vi "Data_filtering_test_2.vi"() -> ()   [LabVIEW 2018]
uses:
  7127b0f4-44e3-4b60-8031-f21aa20547ce.vi
  7127b0f4-44e3-4b60-8031-f21aa20547ce.vi/98f45aaf-d764-4694-8feb-128a91b70d7c.vi
  <vilib>/Analysis/NI_AALBase.lvlib
  <vilib>/Analysis/NI_AALPro.lvlib
panel:
  out "SD speed 2":dbl format="%0.2f"
  out "SD speed 1":dbl format="%0.2f"
  out "SD ideal speed 2":dbl format="%0.2f"
  out "SD ideal speed 1":dbl format="%0.2f"
  out "Speed 2":dbl format="%0.2f"
  out "Speed 1":dbl format="%0.2f"
  out "Ideal speed 2":dbl format="%0.2f"
  out "Ideal speed 1":dbl format="%0.2f"
  out "Proc data":dbl[][](graph)
  out "Speed data":dbl[][](graph)
  in  "Noise SD":dbl=3.0 min=0.0 max=10.0 step=0.1 format="%#_13g"
  out "Noisy raw data":dbl[][](graph)
  out "Pure raw data":dbl[][](graph)
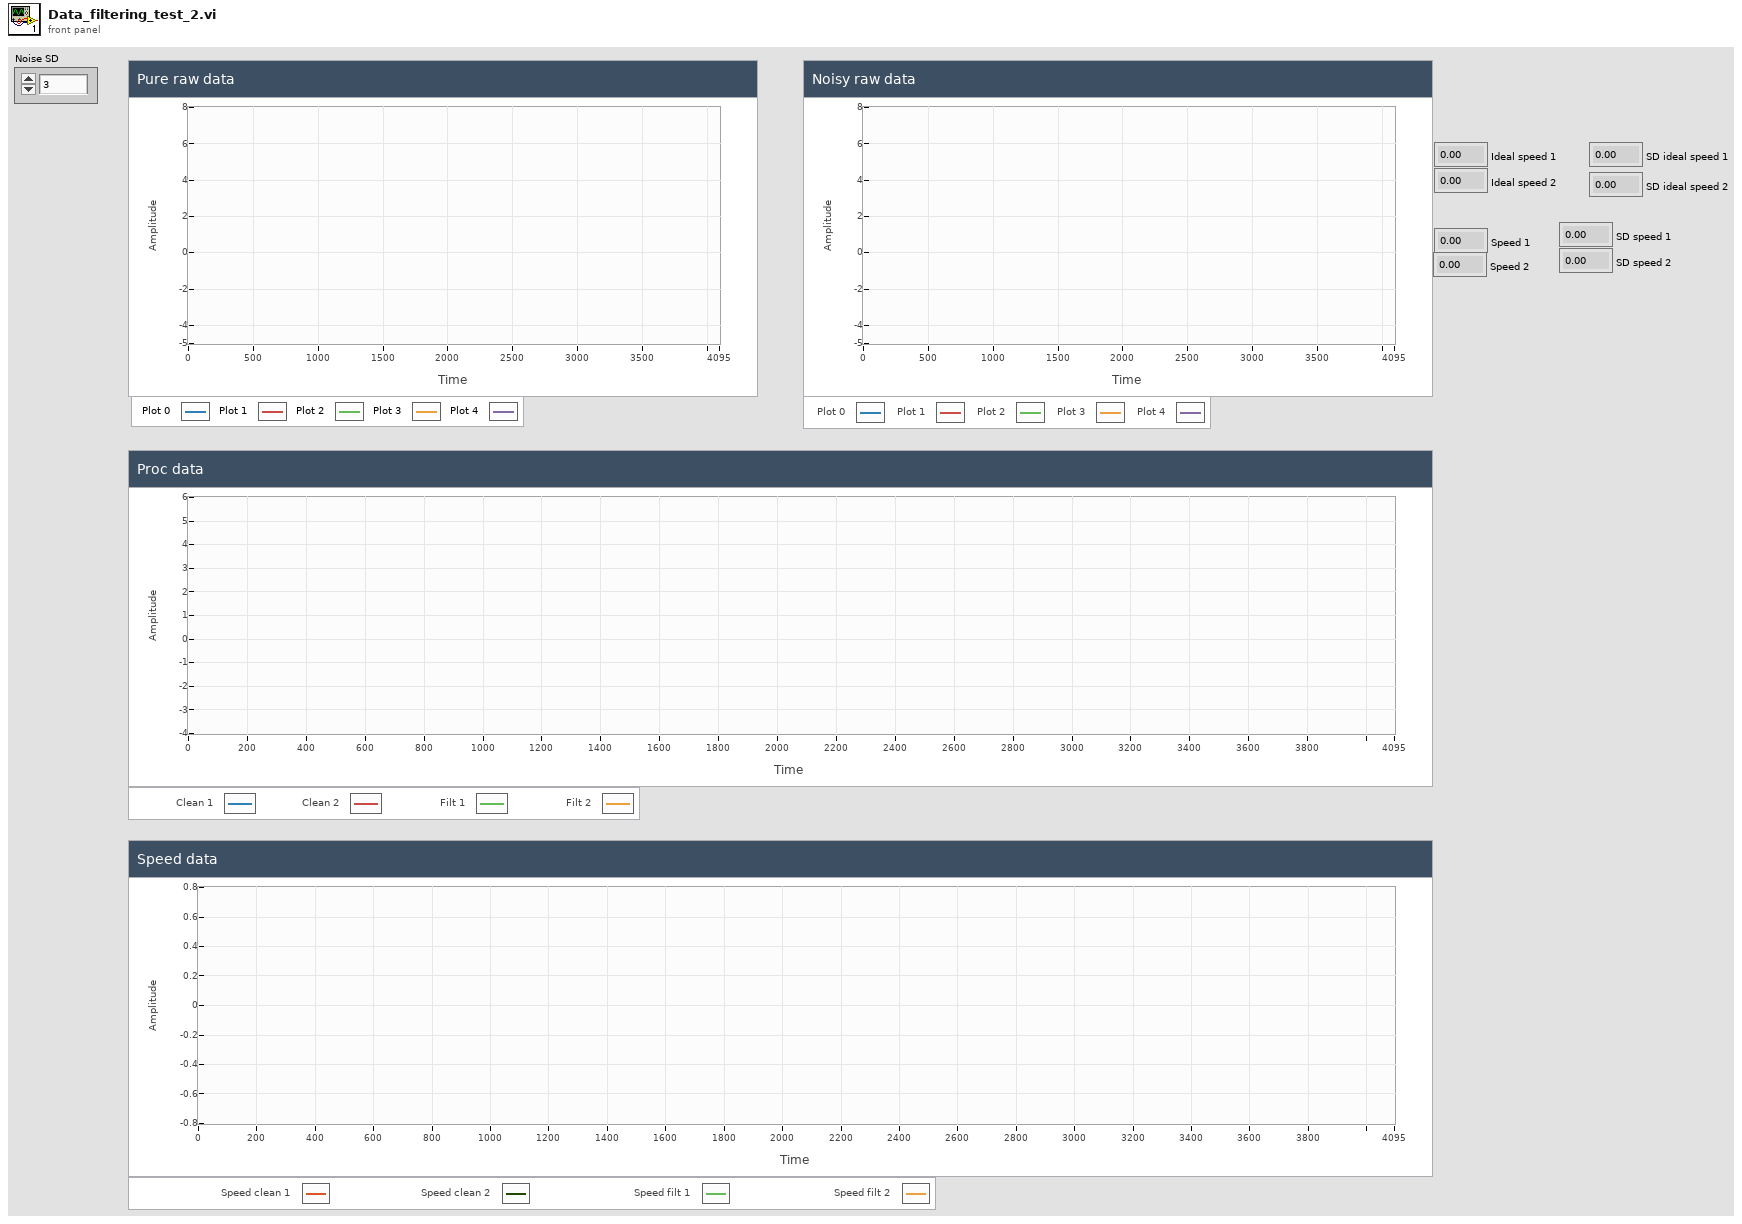
[diagram p1: front panel]
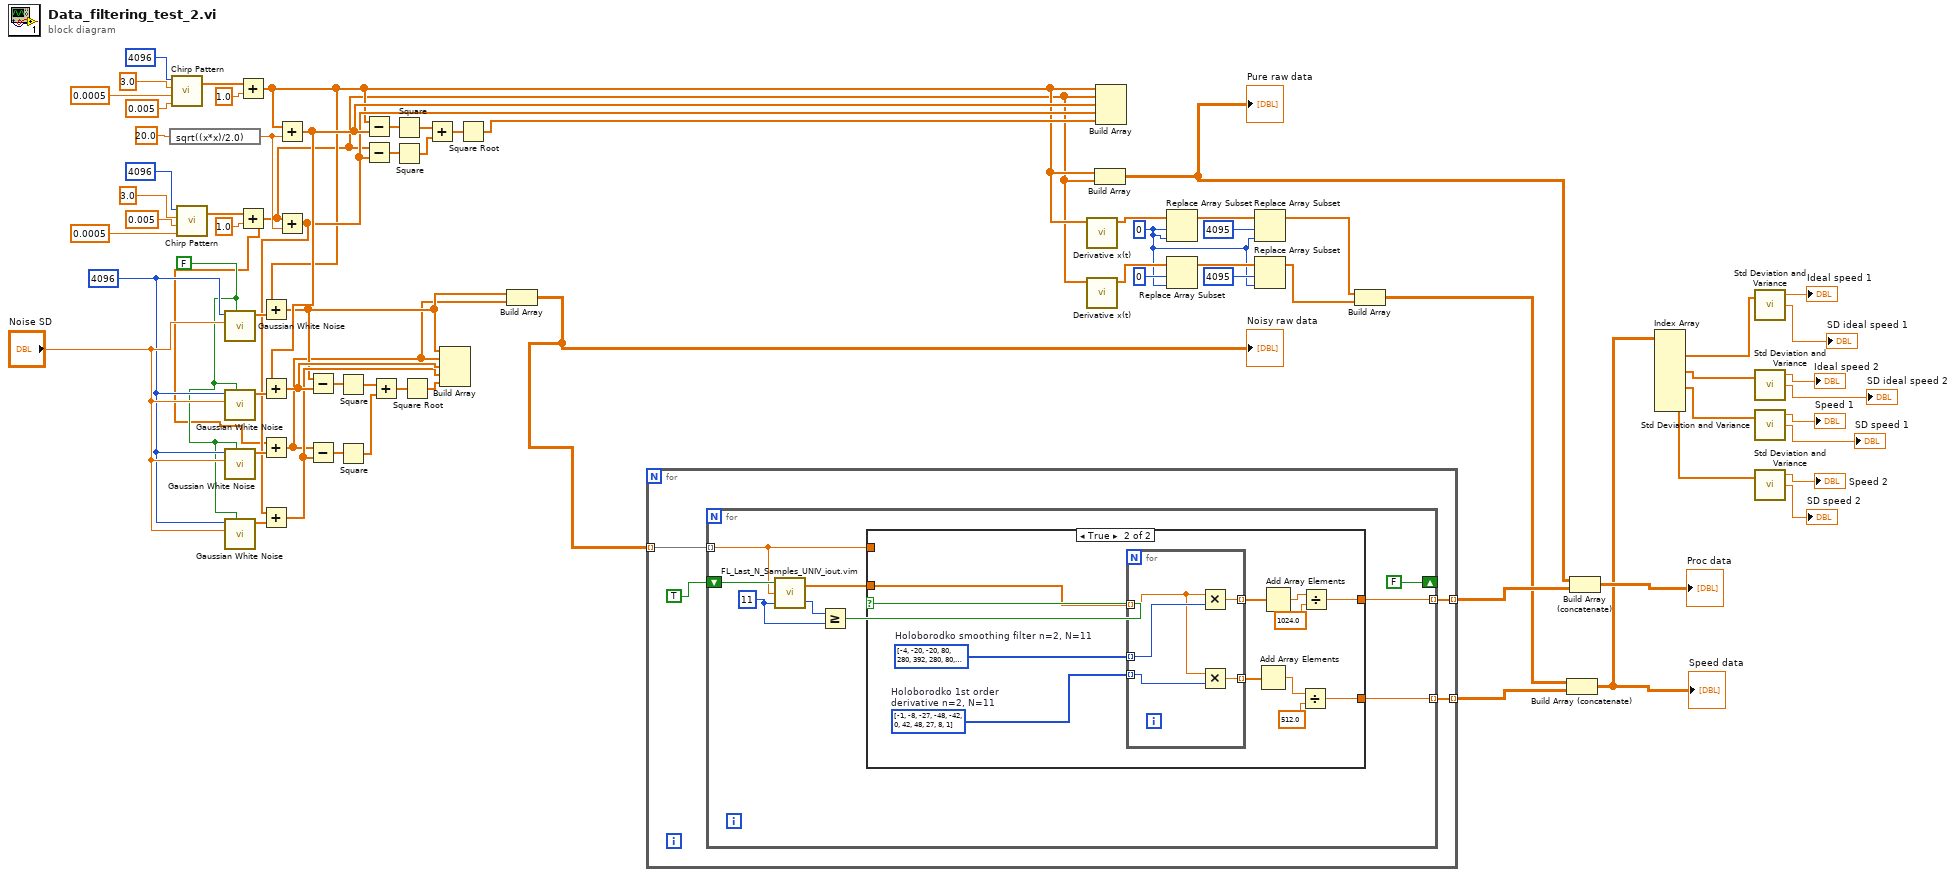
[diagram p0: block diagram]
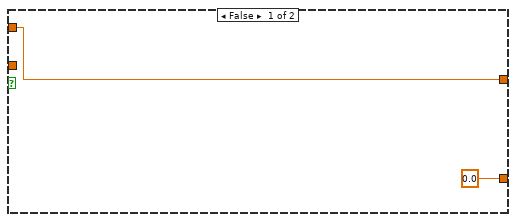
[diagram p2: hidden frame]
diagram:
  w14 = 0 ("index")
  w34 = FALSE ("initialize?")
  w35 = 4096 ("samples")
  n1 = expression code="sqrt((x*x)/2.0)"(20.0) -> (w58:dbl)
  n2 = call <vilib>:"Chirp Pattern.vi"("f2"=0.005, "f1"=0.0005, "amplitude"=3.0, "samples"=4096) -> ("Chirp Pattern"=w67:dbl[])  [unwired: 1 out]
  n3 = call <vilib>:"Chirp Pattern.vi"("f2"=0.0005, "f1"=0.005, "amplitude"=3.0, "samples"=4096) -> ("Chirp Pattern"=w64:dbl[])  [unwired: 1 out]
  n4 = call <vilib>:"Gaussian White Noise.vi"("initialize?"=w34, "standard deviation"="Noise SD", "samples"=w35) -> ("Gaussian noise pattern"=w51:dbl[])  [unwired: 7 in, 1 out]
  n5 = call <vilib>:"Gaussian White Noise.vi"("initialize?"=w34, "standard deviation"="Noise SD", "samples"=w35) -> ("Gaussian noise pattern"=w49:dbl[])  [unwired: 7 in, 1 out]
  n6 = call <vilib>:"Gaussian White Noise.vi"("initialize?"=w34, "standard deviation"="Noise SD", "samples"=w35) -> ("Gaussian noise pattern"=w50:dbl[])  [unwired: 7 in, 1 out]
  n7 = call <vilib>:"Gaussian White Noise.vi"("initialize?"=w34, "standard deviation"="Noise SD", "samples"=w35) -> ("Gaussian noise pattern"=w46:dbl[])  [unwired: 7 in, 1 out]
  n8 = Add(x=w67, y=1.0 ("f2")) -> (x+y=w26:dbl[])
  n9 = Add(x=w64, y=1.0 ("f2")) -> (x+y=w25:dbl[])
  n10 = Add(x=w26, y=w51) -> (x+y=w31:dbl[])
  n11 = Add(x=w25, y=w50) -> (x+y=w30:dbl[])
  n12 = Add(x=w26, y=w58) -> (x+y=w48:dbl[])
  n13 = Add(x=w48, y=w49) -> (x+y=w40:dbl[])
  n14 = Add(x=w25, y=w58) -> (x+y=w47:dbl[])
  n15 = Add(x=w47, y=w46) -> (x+y=w39:dbl[])
  n16 = Subtract(x=w31, y=w40) -> (x-y=w41:dbl[])
  n17 = Subtract(x=w30, y=w39) -> (x-y=w42:dbl[])
  n18 = Square(x=w41) -> (x^2=w43:dbl[])
  n19 = Square(x=w42) -> (x^2=w44:dbl[])
  n20 = Subtract(x=w26, y=w48) -> (x-y=w57:dbl[])
  n21 = Subtract(x=w25, y=w47) -> (x-y=w56:dbl[])
  n22 = Add(x=w43, y=w44) -> (x+y=w45:dbl[])
  n23 = Square(x=w57) -> (x^2=w55:dbl[])
  n24 = Square(x=w56) -> (x^2=w54:dbl[])
  n25 = Square Root(x=w45) -> (sqrt(x)=w38:dbl[])
  n26 = Add(x=w55, y=w54) -> (x+y=w53:dbl[])
  n27 = Build Array(w31, w30, w40, w39, w38) -> ()  [unwired: 1 out]
  n28 = Square Root(x=w53) -> (sqrt(x)=w52:dbl[])
  n29 = Build Array(w31, w30) -> (w29:dbl[][])
  "Noisy raw data" <- w29
  n30 = for {
    tunnel: w29 -> [w74] mode=indexing
    tunnel: [w72] -> w33 mode=indexing
    tunnel: [w71] -> w32 mode=indexing
    n31 = for {
      tunnel: w74 -> [w77] mode=indexing
      shift-right: [FALSE] -> _
      shift-left: TRUE -> [w83]
      tunnel: [w76] -> w72 mode=indexing
      tunnel: [w75] -> w71 mode=indexing
      w80 = 11 ("Buffer length, samples")
      n32 = call "FL_Last_N_Samples_UNIV_iout.vim"("Buffer length, samples"=w80, "Input sample"=w77, "Reset"=w83) -> ("Current buffer length, samples"=w81:i32, "Output Array"=w78:dbl[])
      n33 = Greater Or Equal?(x=w81, y=w80) -> (x >= y?=w79:bool)
      n34 = case shown="True" w79 {
        tunnel: w78 -> [_ w96]
        tunnel: w77 -> [w85 _]
        tunnel: [w85 w87] -> w76
        tunnel: [0.0 w86] -> w75
        frame False {
        }
        frame True {
          w94 = i32[] [-1, -8, -27, -48, -42, 0, 42, 48, 27, 8, 1]  # Holoborodko 1st order derivative n=2, N=11
          w95 = i32[] [-4, -20, -20, 80, 280, 392, 280, 80, -20, -20, -4]  # Holoborodko smoothing filter n=2, N=11
          n35 = for {
            tunnel: w96 -> [w100] mode=indexing
            tunnel: w95 -> [w101] mode=indexing
            tunnel: w94 -> [w99] mode=indexing
            tunnel: [w98] -> w93 mode=indexing
            tunnel: [w97] -> w92 mode=indexing
            n36 = Multiply(x=w100, y=w101) -> (x*y=w98:dbl)
            n37 = Multiply(x=w100, y=w99) -> (x*y=w97:dbl)
          }
          n38 = Add Array Elements(numeric array=w92) -> (sum=w91:dbl)
          n39 = Add Array Elements(numeric array=w93) -> (sum=w88:dbl)
          n40 = Divide(x=w91, y=512.0) -> (x/y=w86:dbl)
          n41 = Divide(x=w88, y=1024.0) -> (x/y=w87:dbl)
        }
      }
    }
  }
  n42 = call <vilib>:"Derivative x(t).vi"("X"=w26) -> ("dX/dt"=w23:dbl[])  [unwired: 9 in, 1 out]
  n43 = call <vilib>:"Derivative x(t).vi"("X"=w25) -> ("dX/dt"=w22:dbl[])  [unwired: 9 in, 1 out]
  n44 = Build Array(w26, w25) -> (w27:dbl[][])
  "Pure raw data" <- w27
  n45 = Build Array(w26, w25, w48, w47, w52) -> ()  [unwired: 1 out]
  n46 = Replace Array Subset(array=w23, new element=w14, index=w14) -> (w18:dbl[])
  n47 = Replace Array Subset(array=w22, new element=w14, index=0) -> (w17:dbl[])
  n48 = Replace Array Subset(array=w18, new element=w14, index=4095) -> (w16:dbl[])
  n49 = Replace Array Subset(array=w17, new element=w14, index=4095) -> (w15:dbl[])
  n50 = Build Array(w16, w15) -> (w24:dbl[][])
  n51 = Build Array (concatenate)(w24, w32) -> (w13:dbl[][])
  "Speed data" <- w13
  n52 = Build Array (concatenate)(w27, w33) -> (→"Proc data":dbl[][])
  n53 = Index Array(array=w13) -> (element #1=w12:dbl[], element #2=w9:dbl[], element #3=w7:dbl[], element #4=w5:dbl[])  [unwired: 8 in]
  n54 = call <vilib>:"Std Deviation and Variance.vi"("X"=w12) -> ("mean"=→"Ideal speed 1":dbl, "standard deviation"=→"SD ideal speed 1":dbl)  [unwired: 1 in, 1 out]
  n55 = call <vilib>:"Std Deviation and Variance.vi"("X"=w9) -> ("mean"=→"Ideal speed 2":dbl, "standard deviation"=→"SD ideal speed 2":dbl)  [unwired: 1 in, 1 out]
  n56 = call <vilib>:"Std Deviation and Variance.vi"("X"=w7) -> ("mean"=→"Speed 1":dbl, "standard deviation"=→"SD speed 1":dbl)  [unwired: 1 in, 1 out]
  n57 = call <vilib>:"Std Deviation and Variance.vi"("X"=w5) -> ("mean"=→"Speed 2":dbl, "standard deviation"=→"SD speed 2":dbl)  [unwired: 1 in, 1 out]
